vi "Stream Too Many Errors Error.vi"(8 "error in (no error)":errorcluster) -> (0 "error out":errorcluster)   [LabVIEW 2020, in "Camera.lvclass"]
uses:
  Camera.lvclass
  Camera.lvclass/Camera.ctl
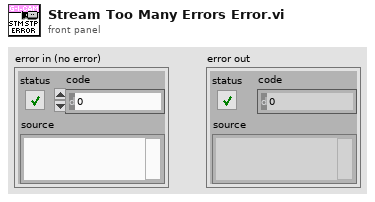
[diagram p1: front panel]
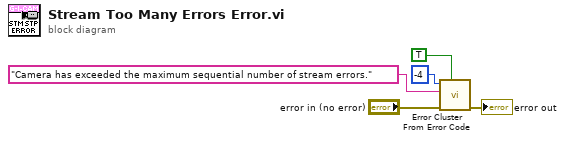
[diagram p0: block diagram]
diagram:
  n1 = call <vilib>:"Error Cluster From Error Code.vi"("show call chain? (False)"=TRUE, "error in (no error)"="error in (no error)", "error message (\"\")"="Camera has exceeded the maximum sequential number of stream errors." ("error message (\"\")"), "error code (0)"=-4) -> ("error out"=→"error out":errorcluster)  [unwired: 5 in]
